vi "test Read Configuration.vi"(8 "error in":errorcluster, 11 "TestCase in":refnum<class "Scripting.lvclass">) -> (0 "error out":errorcluster, 3 "TestCase out":refnum<class "Scripting.lvclass">)   [LabVIEW 2020, in "Scripting.lvclass"]
uses:
  Scripting.lvclass
  <vilib>/addons/_JKI Toolkits/VI Tester/TestCase.llb/TestCase.lvclass
  Scripting/AIM MIL-STD-1553 Scripting.lvlib
  Shared/Address.ctl
  Shared/Message Type.ctl
  Shared/Terminal Endpoint.ctl
  Shared/Parameter Definition.ctl
  Shared/Message Definition.ctl
  Shared/1553 Channel.ctl
  Shared/Minor Frame Definition.ctl
  Shared/Major Frame Definition.ctl
  C:/dev/git/niveristand-custom-device-testing-tools/VeriStandScriptingTestCase/VeriStandScriptingTestCase.lvclass
  C:/Program Files (x86)/National Instruments/LabVIEW 2020/vi.lib/addons/_JKI Toolkits/VI Tester/TestCase.llb/TestCase.lvclass
  C:/dev/git/niveristand-aim-milStd1553-custom-device/Source/Custom Device Support/Tests/Unit/Scripting/Scripting.lvclass
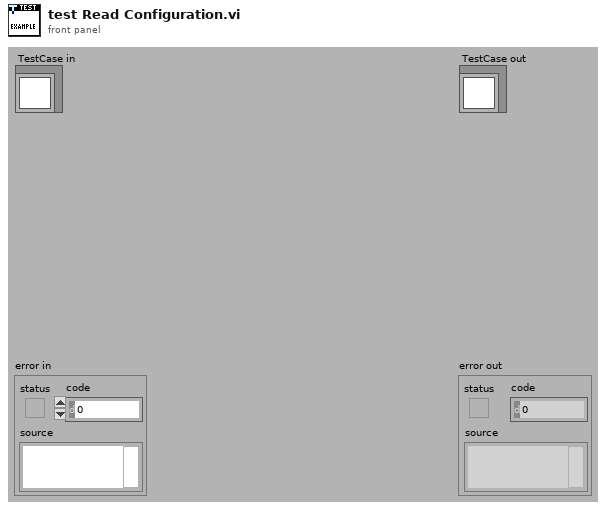
[diagram p1: front panel]
types:
  T1 = typedef "1553 Channel.ctl" = cluster{"HW channel":u16, "terminal addresses":T2[], "terminal names":string[], "acyclic frame names":string[], "major frames":T3[], "minor frames":T4[], "messages":T5[]}
  T2 = typedef "Address.ctl" = u16
  T3 = typedef "Major Frame Definition.ctl" = cluster{"name":string, "minor frames":string[]}
  T4 = typedef "Minor Frame Definition.ctl" = cluster{"name":string, "messages":string[]}
  T5 = typedef "Message Definition.ctl" = cluster{"name":string, "message type":T6, "endpoint Tx":T7, "endpoint Rx":T7, "create timestamp channel":bool, "mode code":u16, "number of words":u16, "parameters":cluster{"name":string, "default value":dbl, "unit":string, "parameter definition":T8}[]}
  T6 = typedef "Message Type.ctl" = string
  T7 = typedef "Terminal Endpoint.ctl" = cluster{"terminal address":T2, "subaddress":T2}
  T8 = typedef "Parameter Definition.ctl" = cluster{"start index":i32, "size (bits)":i32, "encoding":enum16{"BNR", "BCD", "Discrete"}, "signed":bool, "multiplier":dbl, "offset":dbl}
  T9 = typedef "Custom Device API.lvlib/Custom Device Item Ref.ctl" = u64
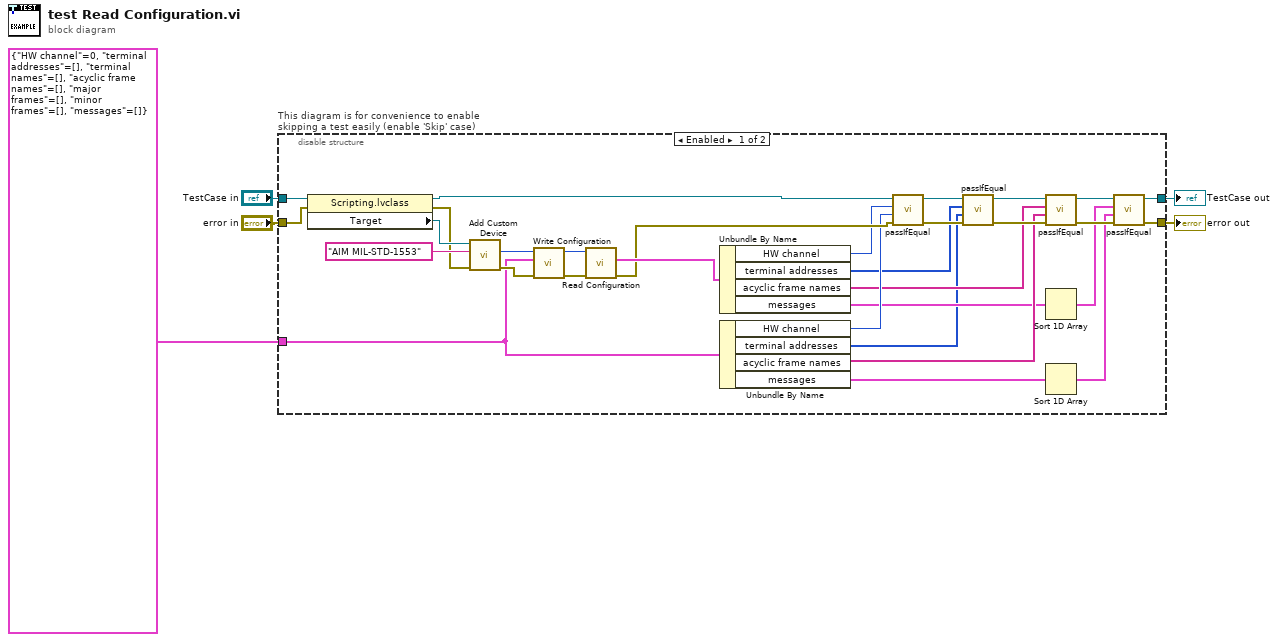
[diagram p0: block diagram]
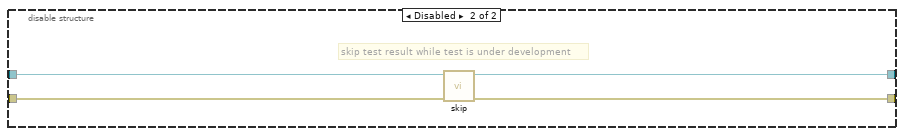
[diagram p2: hidden frame]
diagram:
  n1 = disable-structure "This diagram is for convenience to enable skipping a test easily (enable 'Skip' case)" shown="Enabled" {
    disable-tunnel: "TestCase in" -> [w35 w40]
    disable-tunnel: [w13 w38] -> w2
    disable-tunnel: [w14 w39] -> w4
    disable-tunnel: "error in" -> [w31 w37]
    disable-tunnel: T1 {"HW channel"=0, "terminal addresses"=[], "terminal names"=[], "acyclic frame names"=[], "major frames"=[], "minor frames"=[], "messages"=[]} -> [w6 _]
    frame Enabled {
      n2 = property class="Scripting.lvclass"(reference=w35, error in=w31) -> (reference out=w29:refnum<class "Scripting.lvclass">, error out=w30:errorcluster, "Target"=w34:refnum<k24>)
      n3 = call "Add Custom Device.vi"("error in"=w30, "name"="AIM MIL-STD-1553", "target in"=w34) -> ("error out"=w32:errorcluster, "Ballard MIL-STD 1553 custom device"=w33:T9)  [unwired: 6 in, 1 out]
      n4 = call "Write Configuration.vi"("error in"=w32, "1553 configuration"=w6, "custom device ref"=w33) -> ("error out"=w27:errorcluster, "custom device ref out"=w28:T9)  [unwired: 7 in]
      n5 = call "Read Configuration.vi"("error in"=w27, "custom device ref"=w28) -> ("error out"=w25:errorcluster, "1553 configuration out"=w26:T1)  [unwired: 7 in, 1 out]
      n6 = Unbundle By Name(w26) -> ("HW channel"=w19:u16, "terminal addresses"=w8:T2[], "acyclic frame names"=w17:string[], "messages"=w11:T5[])
      n7 = Unbundle By Name(w6) -> ("HW channel"=w20:u16, "terminal addresses"=w7:T2[], "acyclic frame names"=w18:string[], "messages"=w12:T5[])
      n8 = call-dynamic "passIfEqual.vi"("error in (no error)"=w25, "y"=w20, "x"=w19, "TestCase in"=w29) -> ("error out"=w23:errorcluster, "TestCase out"=w24:refnum<class "Scripting.lvclass">)  [unwired: 6 in]
      n9 = call-dynamic "passIfEqual.vi"("error in (no error)"=w23, "y"=w7, "x"=w8, "TestCase in"=w24) -> ("error out"=w21:errorcluster, "TestCase out"=w22:refnum<class "Scripting.lvclass">)  [unwired: 6 in]
      n10 = call-dynamic "passIfEqual.vi"("error in (no error)"=w21, "y"=w18, "x"=w17, "TestCase in"=w22) -> ("error out"=w16:errorcluster, "TestCase out"=w15:refnum<class "Scripting.lvclass">)  [unwired: 6 in]
      n11 = Sort 1D Array(array=w11) -> (sorted array=w10:T5[])
      n12 = Sort 1D Array(array=w12) -> (sorted array=w9:T5[])
      n13 = call-dynamic "passIfEqual.vi"("error in (no error)"=w16, "y"=w9, "x"=w10, "TestCase in"=w15) -> ("error out"=w14:errorcluster, "TestCase out"=w13:refnum<class "Scripting.lvclass">)  [unwired: 6 in]
    }
    frame Disabled {
      # "skip test result while test is under development"
      n14 = call <vilib>:"skip.vi"("error in (no error)"=w37, "TestCase in"=w40) -> ("error out"=w39:errorcluster, "TestCase out"=w38:refnum<class "Scripting.lvclass">)  [unwired: 8 in]
    }
  }
  "error out" <- w4
  "TestCase out" <- w2
